vi "App_tau delay.vi"(0 "reference in":refnum<class "Fcurve.lvclass">, 5 "error in (no error)":errorcluster) -> (14 "reference out":refnum<class "Fcurve.lvclass">, 16 "# of samples":i32, 19 "error out":errorcluster)   [LabVIEW 2019, in "Fcurve.lvclass"]
doc: "This takes to account the delay time of the slowest time constant of the afm control system"
uses:
  Fcurve.lvclass
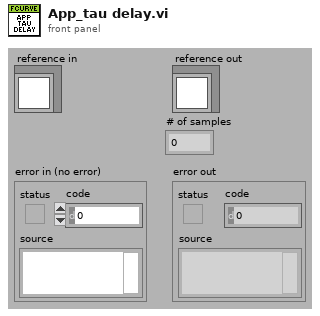
[diagram p1: front panel]
types:
  T1 = typedef "Fcurve.lvclass/ObjectAttributes.ctl" = cluster{"MyAttribute":dbl, "Fcurve Metadata":T2, "Contact Spread of dev":dbl, "Tau Delay (ms)":dbl, "Points of contact":dbl, "Def_wfm":cluster{"Max":dbl, "Min":dbl}, "Zpos_wfm":cluster{"Max":dbl, "Min":dbl}, "Contact stat?":bool, "Real AI dt (s)":dbl, "Decimation":cluster{"App":cluster{"Dec":i32, "apply":bool}, "Con":cluster{"Dec":i32, "apply":bool}, "Ret":cluster{"Dec":i32, "apply":bool}}, "Segment def[0]":dbl, "Segment Zpos[0]":dbl, "Raw Datum":waveform(dbl)[], "Group metadata":T3, "M_data obj":refnum<class "metadata.lvclass">, "Channel name(s)":string[], "Segment fcurve data":cluster{"X":dbl[], "Y":dbl[]}[], "Segment duration":cluster{"Start":i32, "Duration":i32}[], "Segment info":T4[], "Segment durations (S)":dbl[], "Segments Maxmin":T6[]}
  T2 = typedef "Fcurve.lvclass/Metadata.ctl" = cluster{"dt (us)":dbl, "Dec Factor":dbl, "Z piezo Sensitivity (nm/V)":dbl, "K (N/m)":dbl, "Sp (V)":dbl, "Contact (ms)":dbl, "Zpos contact":dbl, "Vel_app (nm/s)":dbl, "Vel_ret (nm/s)":dbl, "deltaV (nm)":dbl, "Def_V0 (v)":dbl, "Piezo gain":dbl, "invOLS (nm/V)":dbl}
  T3 = typedef "TDMS_DataHandler.lvclass/Fcurve Meta data.ctl" = cluster{"property names":string[], "property values":variant[]}
  T4 = typedef "Fcurve.lvclass/Fcurve segments --cluster.ctl" = cluster{"type":T5, "nb points":i32, "dec factor":u32, "sampling rate (S/s)":u32}
  T5 = typedef "metadata.lvclass/Segment type--combobox.ctl" = string
  T6 = typedef "Fcurve.lvclass/Segment MaxMin --cluster.ctl" = cluster{"Def":cluster{"max value":dbl, "min value":dbl}, "Zpos":cluster{"max value":dbl, "min value":dbl}}
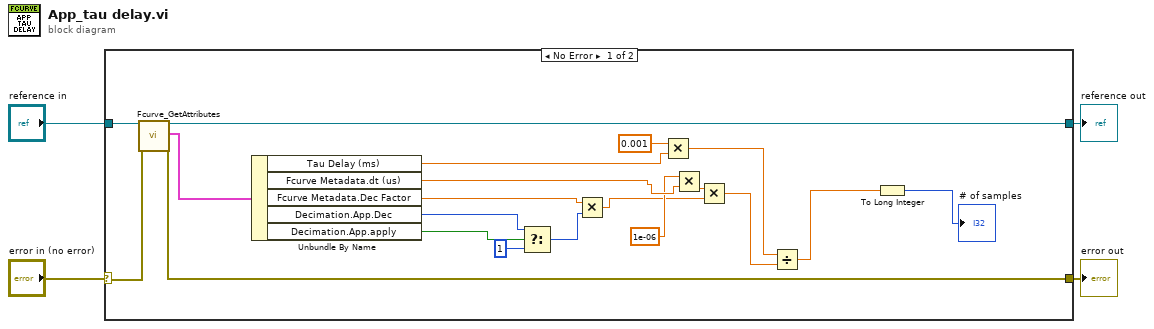
[diagram p0: block diagram]
diagram:
  n1 = case shown="No Error" "error in (no error)" {
    selector: "error in (no error)" -> [w22 w26]
    tunnel: [w21 w26] -> w3
    tunnel: [w23 w25] -> w1
    tunnel: "reference in" -> [w24 w25]
    frame No Error {
      n2 = call "Fcurve_GetAttributes.vi"("reference in"=w24, "error in (no error)"=w22) -> ("reference out"=w23:refnum<class "Fcurve.lvclass">, "attributes"=w20:T1, "error out"=w21:errorcluster)  [unwired: 14 in, 1 out]
      n3 = Unbundle By Name(w20) -> ("Tau Delay (ms)"=w18:dbl, "Fcurve Metadata.dt (us)"=w15:dbl, "Fcurve Metadata.Dec Factor"=w12:dbl, "Decimation.App.Dec"=w7:i32, "Decimation.App.apply"=w8:bool)
      n4 = Select(t=w7, s=w8, f=1) -> (s? t:f=w5:i32)
      n5 = Multiply(x=w12, y=w5) -> (x*y=w11:dbl)
      n6 = Multiply(x=0.001, y=w18) -> (x*y=w16:dbl)
      n7 = Multiply(x=1e-06, y=w15) -> (x*y=w13:dbl)
      n8 = Multiply(x=w13, y=w11) -> (x*y=w19:dbl)
      n9 = Divide(x=w16, y=w19) -> (x/y=w10:dbl)
      n10 = To Long Integer(number=w10) -> (32bit integer=→"# of samples":i32)
    }
    frame Error {
    }
  }
  "error out" <- w3
  "reference out" <- w1
